vi "loadDeviceName.vi"(8 "error in (no error)":errorcluster, 10 "NativeXML in":refnum<class "NativeXML.lvclass">, 11 "deviceDataBase in":refnum<class "deviceDataBase.lvclass">) -> (0 "error out":errorcluster, 1 "deviceName":string, 2 "NativeXML out":refnum<class "NativeXML.lvclass">, 3 "deviceDataBase out":refnum<class "deviceDataBase.lvclass">)   [LabVIEW 2009, in "Tools.lvlib" / "DatabaseHelpers.lvlib" / "deviceDataBase.lvclass"]
uses:
  deviceDataBase.lvclass
  NativeXML/NativeXML.lvclass
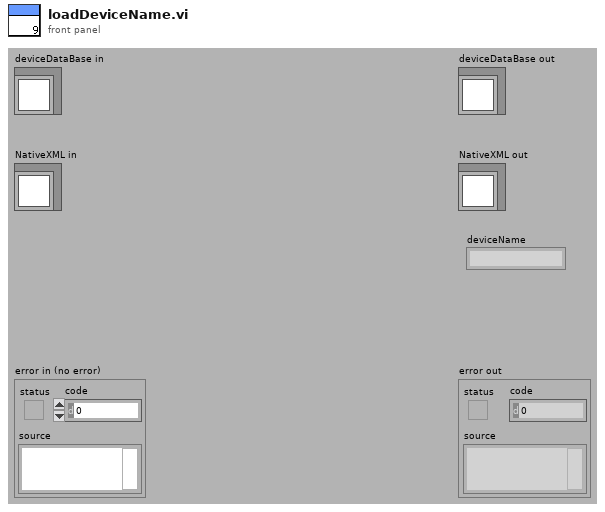
[diagram p1: front panel]
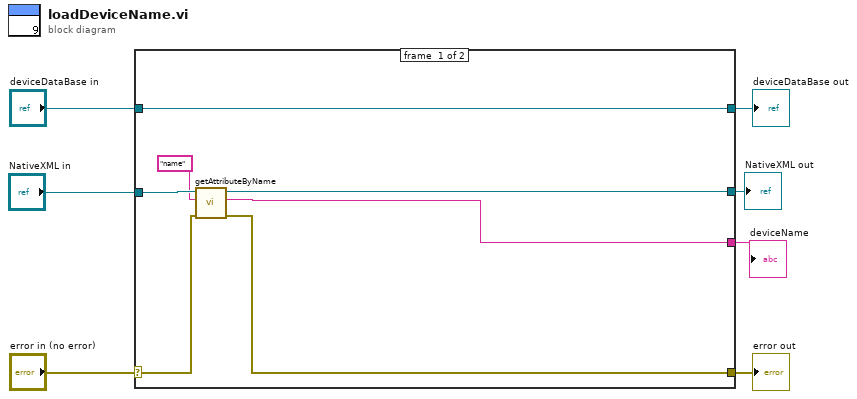
[diagram p0: block diagram]
diagram:
  n1 = case shown="No Error" "error in (no error)" {
    selector: "error in (no error)" -> [w9 w16]
    tunnel: [w10 w16] -> w6
    tunnel: [w14 w15] -> w4
    tunnel: "deviceDataBase in" -> [w14 w15]
    tunnel: "NativeXML in" -> [w13 _]
    tunnel: [w12 _] -> w2
    tunnel: [w11 _] -> w1
    frame #0 {
      n2 = call "getAttributeByName.vi"("error in (no error)"=w9, "name"="name", "NativeXML in"=w13) -> ("error out"=w10:errorcluster, "Attribute String"=w11:string, "NativeXML out"=w12:refnum<class "NativeXML.lvclass">)  [unwired: 6 in]
    }
    frame #1 {
    }
  }
  "error out" <- w6
  "deviceDataBase out" <- w4
  "NativeXML out" <- w2
  "deviceName" <- w1
